vi "Save Configuration.vi"(8 "error in (no error)":errorcluster, 11 "Report Generator in":refnum<class "Report Generator.lvclass">) -> (0 "error out":errorcluster, 3 "Report Generator out":refnum<class "Report Generator.lvclass">)   [LabVIEW 2020, in "Report Generator.lvclass"]
uses:
  Report Generator.lvclass
  Application Framework/Process Classes/Process/Process.lvclass
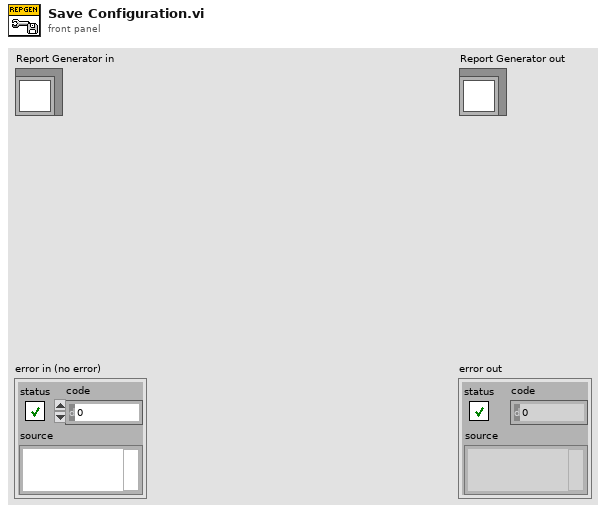
[diagram p1: front panel]
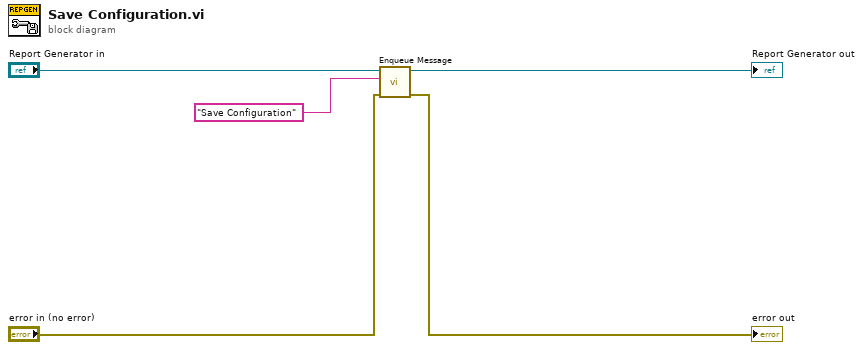
[diagram p0: block diagram]
diagram:
  n1 = call "Enqueue Message.vi"("error in (no error)"="error in (no error)", "Message"="Save Configuration", "Process In"="Report Generator in") -> ("error out"=→"error out":errorcluster, "Process Out"=→"Report Generator out":refnum<class "Report Generator.lvclass">)  [unwired: 7 in]
